vi "Test keyence.vi"() -> ()   [LabVIEW 2023]
panel:
  out "ASCII QR Code":string
  out "error out 2":errorcluster
  out "error out":errorcluster
  in  "Port":u16
  in  "IP address":string
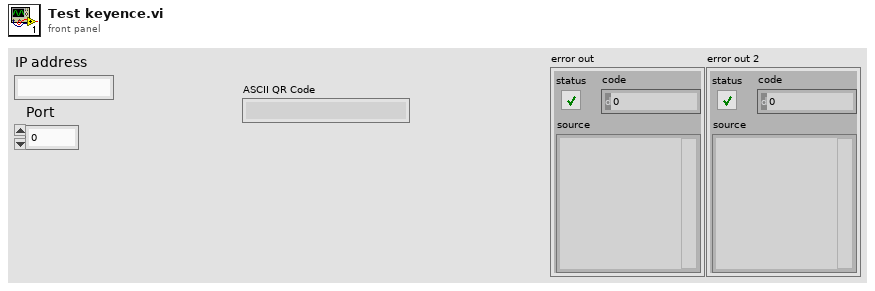
[diagram p1: front panel]
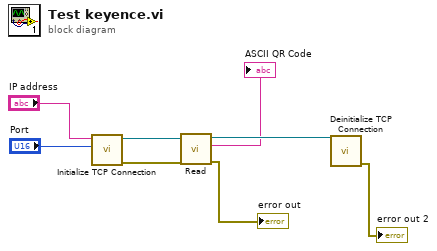
[diagram p0: block diagram]
diagram:
  n1 = call "Initialize TCP Connection.vi"("Port"="Port", "IP address"="IP address") -> ("error out"=w5:errorcluster, "TCP Network Connection out"=w6:refnum<k5>)  [unwired: 8 in]
  n2 = call "Read.vi"("error in"=w5, "TCP in"=w6) -> ("error out"=→"error out":errorcluster, "ASCII QR Code"=→"ASCII QR Code":string, "TCP Network Connection out"=w4:refnum<k5>)  [unwired: 7 in]
  n3 = call "Deinitialize TCP Connection.vi"("TCP Network Connection in"=w4) -> ("error out"=→"error out 2":errorcluster)  [unwired: 10 in]
